vi "NI9205.vi"() -> ()   [LabVIEW 2019]
panel:
  out "AI1 - AI9":dbl
  out "AI9":dbl
  out "AI1":dbl
  out "AI0 - AI8":dbl
  out "AI8":dbl
  out "AI0":dbl
  out "DAQ Anolog Input Signals (Array)":dbl[](array[numeric])
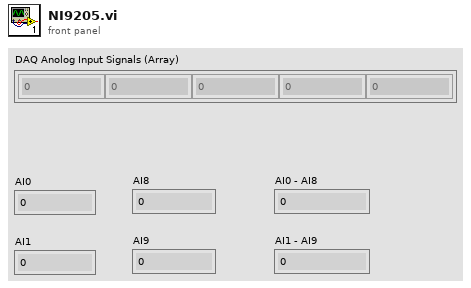
[diagram p1: front panel]
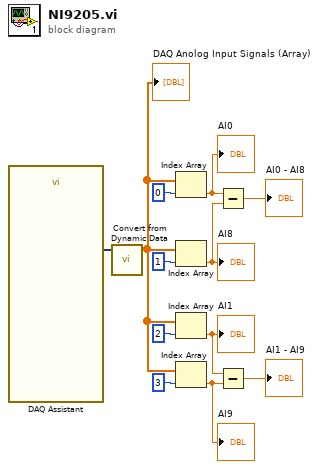
[diagram p0: block diagram]
diagram:
  n1 = call "DAQ Assistant"() -> ("data"=w12:dynamicdata)  [unwired: 17 in, 2 out]
  n2 = call "Convert from Dynamic Data"("Dynamic Data Type"=w12) -> ("Array"=w4:dbl[])  [unwired: 3 in]
  "DAQ Anolog Input Signals (Array)" <- w4
  n3 = Index Array(array=w4, index=0) -> (element=w9:dbl)
  "AI0" <- w9
  n4 = Index Array(array=w4, index=1) -> (element=w8:dbl)
  "AI8" <- w8
  n5 = Index Array(array=w4, index=2) -> (element=w2:dbl)
  "AI1" <- w2
  n6 = Index Array(array=w4, index=3) -> (element=w1:dbl)
  "AI9" <- w1
  n7 = Subtract(x=w9, y=w8) -> (x-y=→"AI0 - AI8":dbl)
  n8 = Subtract(x=w2, y=w1) -> (x-y=→"AI1 - AI9":dbl)
